vi "Write Config.vi"(8 "error in (no error)":errorcluster, 10 "Config":T1, 11 "Path":path) -> (0 "error out":errorcluster)   [LabVIEW 2020, in "MacroAssert.lvlib"]
doc: "Writes to a config file located at <B>Path</B>."
uses:
  MacroAssert.lvlib
  <vilib>/Utility/config.llb/NI_LVConfig.lvlib
  <vilib>/Utility/config.llb/Write Key (String).vi
  <vilib>/Utility/config.llb/Write Key (Boolean).vi
  31d934df-4868-4a69-9c54-9262212b3b47.vi
  CTLs/Config Key.ctl
  CTLs/Config.ctl
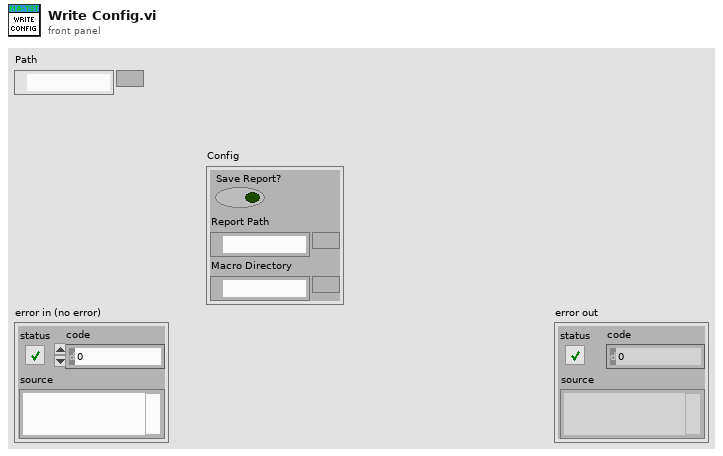
[diagram p1: front panel]
types:
  T1 = typedef "MacroAssert.lvlib/Config.ctl" = cluster{"Save Report?":bool, "Report Path":path, "Macro Directory":path}
  T2 = typedef "MacroAssert.lvlib/Config Key.ctl" = enum16{"SaveReport", "ReportPath", "MacroDirectory"}
  T3 = typedef "NI_LVConfig.lvlib/Config Data RefNum.ctl" = refnum<k1>
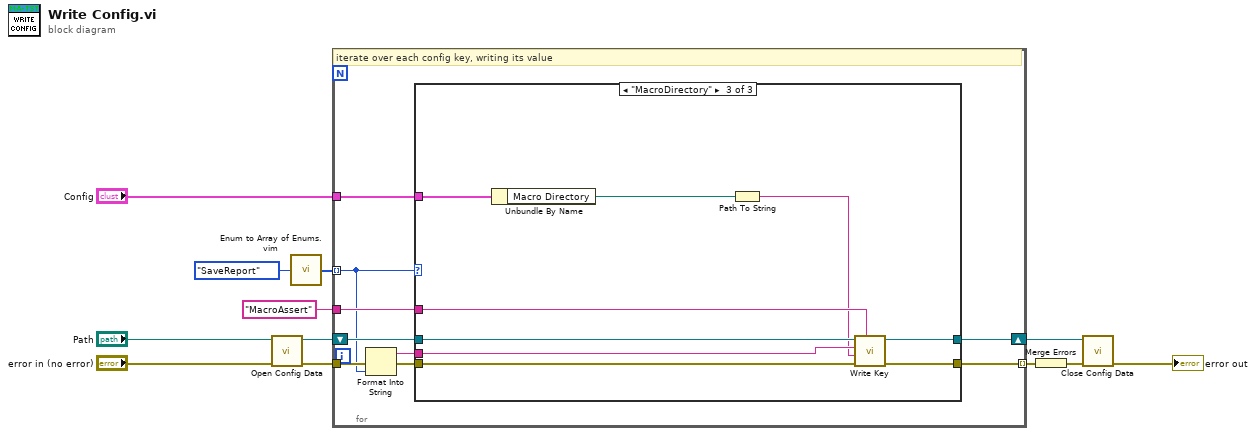
[diagram p0: block diagram]
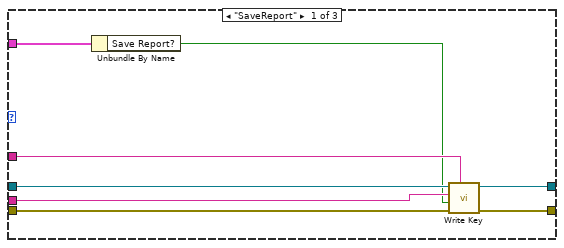
[diagram p2: hidden frame]
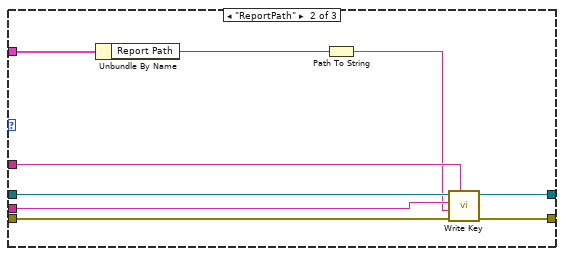
[diagram p3: hidden frame]
diagram:
  n1 = call <vilib>:"Open Config Data.vi"("error in (no error)"="error in (no error)", "configuration file path"="Path") -> ("error out"=w11:errorcluster, "refnum"=w12:T3)  [unwired: 7 in, 1 out]
  n2 = call "Enum to Array of Enums.vim"("enum"=Config_Key."SaveReport" ("Config Key")) -> ("array of enums"=w9:T2[])
  n3 = for {
    tunnel: w9 -> [w16] mode=indexing
    tunnel: "MacroAssert" ("section") -> [w17]
    tunnel: [w14] -> w7 mode=indexing
    tunnel: w11 -> [w21]
    shift-right: [w15] -> w6
    shift-left: w12 -> [w18]
    tunnel: "Config" -> [w19]
    # "iterate over each config key, writing its value"
    n4 = Format Into String(error in=w21, w16) -> (resulting string=w13:string, error out=w20:errorcluster)  [unwired: 2 in]
    n5 = case shown="\"MacroDirectory\"" w16 {
      tunnel: w20 -> [w29 w38 w47]
      tunnel: w19 -> [w27 w36 w45]
      tunnel: w18 -> [w28 w37 w46]
      tunnel: w17 -> [w24 w32 w41]
      tunnel: [w26 w35 w44] -> w15
      tunnel: [w25 w34 w43] -> w14
      tunnel: w13 -> [w23 w31 w40]
      frame "SaveReport" {
        n6 = Unbundle By Name(w27) -> ("Save Report?"=w22:bool)
        n7 = call-poly <vilib>:"Write Key.vi"("section"=w24, "error in (no error)"=w29, "value"=w22, "key"=w23, "refnum"=w28) -> ("error out"=w25:errorcluster, "refnum out"=w26:T3)  [unwired: 4 in, 1 out]
      }
      frame "ReportPath" {
        n8 = Unbundle By Name(w36) -> ("Report Path"=w33:path)
        n9 = Path To String(path=w33) -> (string=w30:string)
        n10 = call-poly <vilib>:"Write Key.vi"("section"=w32, "error in (no error)"=w38, "value"=w30, "key"=w31, "refnum"=w37) -> ("error out"=w34:errorcluster, "refnum out"=w35:T3)  [unwired: 4 in, 1 out]
      }
      frame "MacroDirectory" {
        n11 = Unbundle By Name(w45) -> ("Macro Directory"=w42:path)
        n12 = Path To String(path=w42) -> (string=w39:string)
        n13 = call-poly <vilib>:"Write Key.vi"("section"=w41, "error in (no error)"=w47, "value"=w39, "key"=w40, "refnum"=w46) -> ("error out"=w43:errorcluster, "refnum out"=w44:T3)  [unwired: 4 in, 1 out]
      }
    }
  }
  n14 = Merge Errors(w7) -> (w10:errorcluster)
  n15 = call <vilib>:"Close Config Data.vi"("error in (no error)"=w10, "refnum"=w6) -> ("error out"=→"error out":errorcluster)  [unwired: 8 in, 1 out]
